vi "Image_RAW_Get_Timestamp.vi"(8 "error in (no error)":errorcluster, 11 "Frame (U8)":u8[](array[numeric])) -> (0 "error out":errorcluster, 2 "Frame Timestamp":u64)   [LabVIEW 2020]
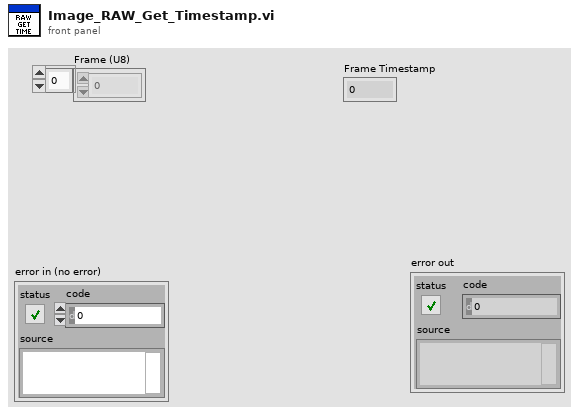
[diagram p1: front panel]
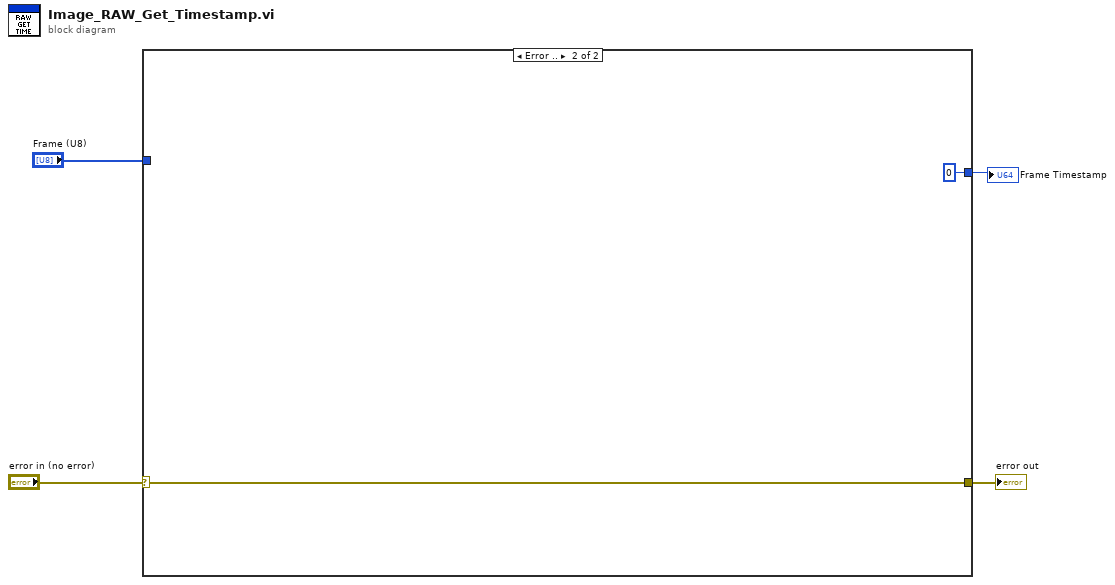
[diagram p0: block diagram]
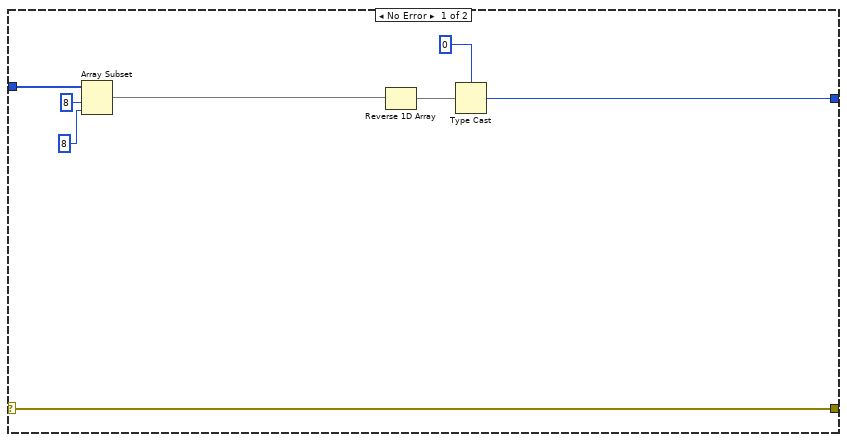
[diagram p2: hidden frame]
diagram:
  n1 = case shown="Error .." "error in (no error)" {
    selector: "error in (no error)" -> [w5 w13]
    tunnel: [w11 u64 0] -> w3
    tunnel: [w5 w13] -> w2
    tunnel: "Frame (U8)" -> [w9 _]
    frame No Error {
      n2 = Array Subset(array=w9, index=8, length=8) -> (w6:u8[])
      n3 = Reverse 1D Array(array=w6) -> (reversed array=w10:u8[])
      n4 = Type Cast(type=u64 0, x=w10) -> (*(type *) &x=w11:u64)
    }
    frame Error {
    }
  }
  "error out" <- w2
  "Frame Timestamp" <- w3
